vi "Voltage_laps.vi"(4 "Sweep 2":T1={"DorG_2"="", "Vvar_2_start"=0.0, "Vvar_2_step"=0.0, "Vvar_2_Stop"=0.0, "Vvar_0_stop 2"=0.0, "DrainCurComp_2 2"=1e-06, "GateCurComp_2 2"=1e-06, "Vvar_2_holdtime 2"=0.0, "Vvar_2_delaytime 2"=0.0, "IntPts_2 2"=100.0, "Set Swe_2_Mode 2"="", "Sweep Spacing_2 2"=""}, 5 "Sweep 1":T2={"DorG_1"="", "Vvar_1_start"=0.0, "Vvar_1_step"=0.0, "Vvar_1_Stop"=0.0, "Vvar_0_stop"=0.0, "DrainCurComp_1"=1e-06, "GateCurComp_1"=1e-06, "Vvar_1_holdtime"=0.0, "Vvar_1_delaytime"=0.0, "IntPts_1"=100.0, "Set Swe_1_Mode"="", "Sweep Spacing_1"=""}, 6 "error in (no error)":errorcluster, 7 "Sweep 2":bool, 8 "smu_1_port":string, 9 "VISA resource name":refnum<visa-resource-name>) -> (0 "error out":errorcluster, 1 "Recorded_data":dbl[][](array[numeric]), 3 "VISA resource name out":refnum<visa-resource-name>)   [LabVIEW 2021]
panel:
  out "V Slave":string
  out "V Lead":string
  # "Single"
  # "Double"
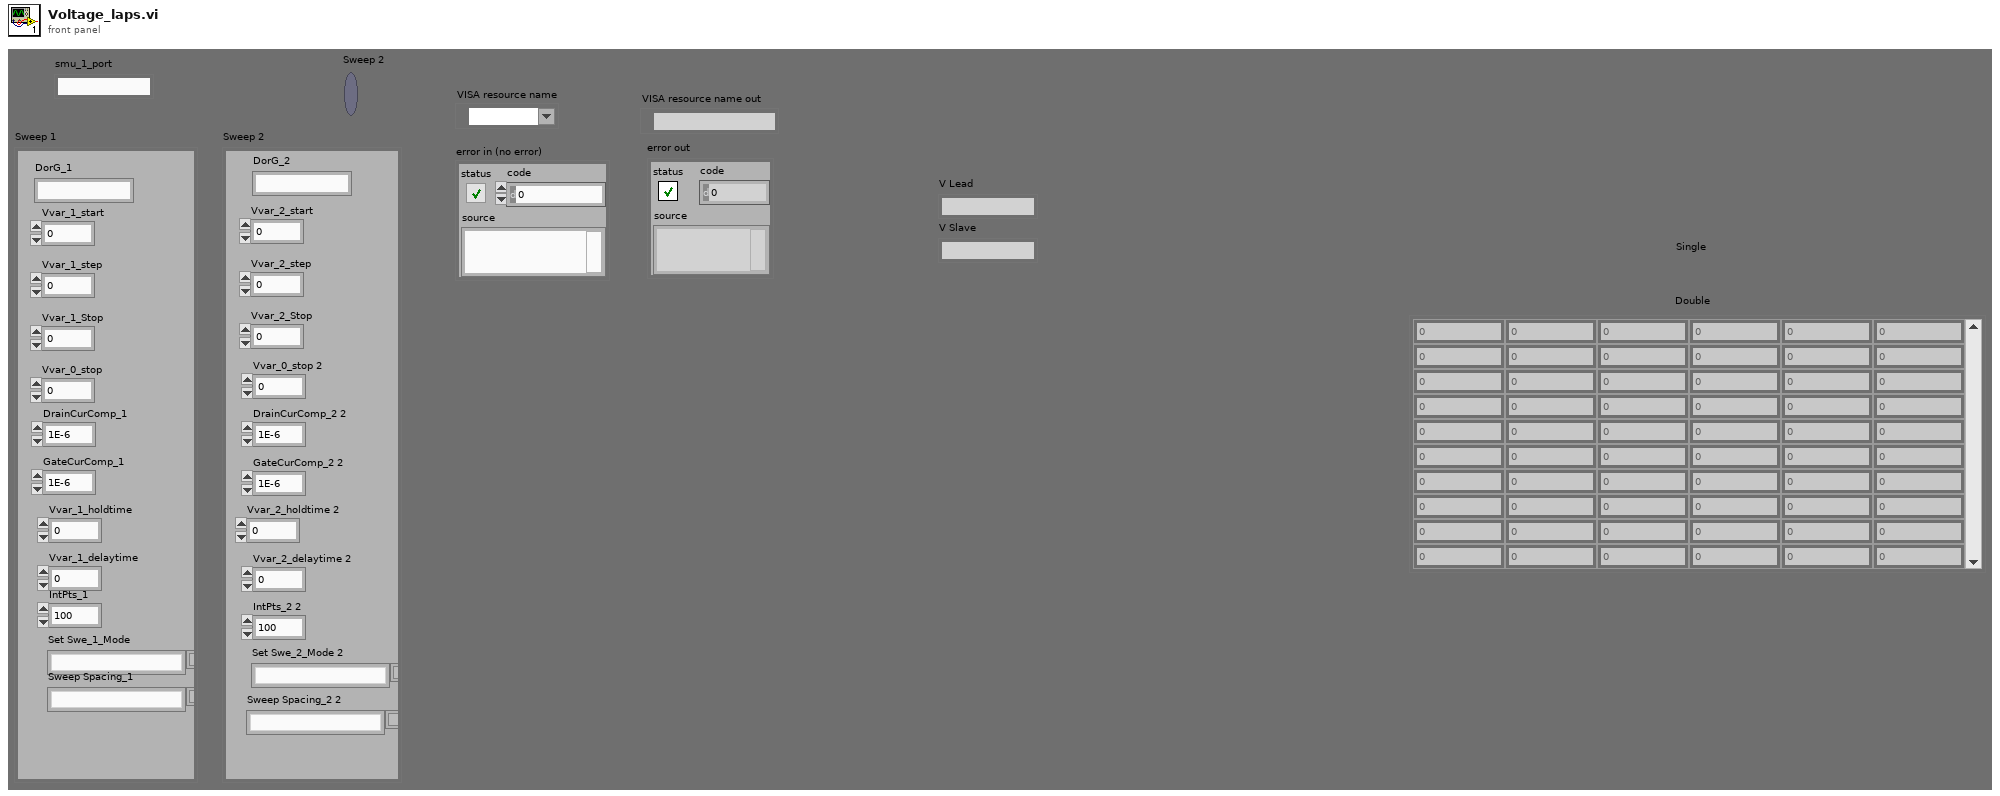
[diagram p1: front panel]
types:
  T1 = cluster{"DorG_2":string, "Vvar_2_start":dbl, "Vvar_2_step":dbl, "Vvar_2_Stop":dbl, "Vvar_0_stop 2":dbl, "DrainCurComp_2 2":dbl, "GateCurComp_2 2":dbl, "Vvar_2_holdtime 2":dbl, "Vvar_2_delaytime 2":dbl, "IntPts_2 2":dbl, "Set Swe_2_Mode 2":string, "Sweep Spacing_2 2":string}
  T2 = cluster{"DorG_1":string, "Vvar_1_start":dbl, "Vvar_1_step":dbl, "Vvar_1_Stop":dbl, "Vvar_0_stop":dbl, "DrainCurComp_1":dbl, "GateCurComp_1":dbl, "Vvar_1_holdtime":dbl, "Vvar_1_delaytime":dbl, "IntPts_1":dbl, "Set Swe_1_Mode":string, "Sweep Spacing_1":string}
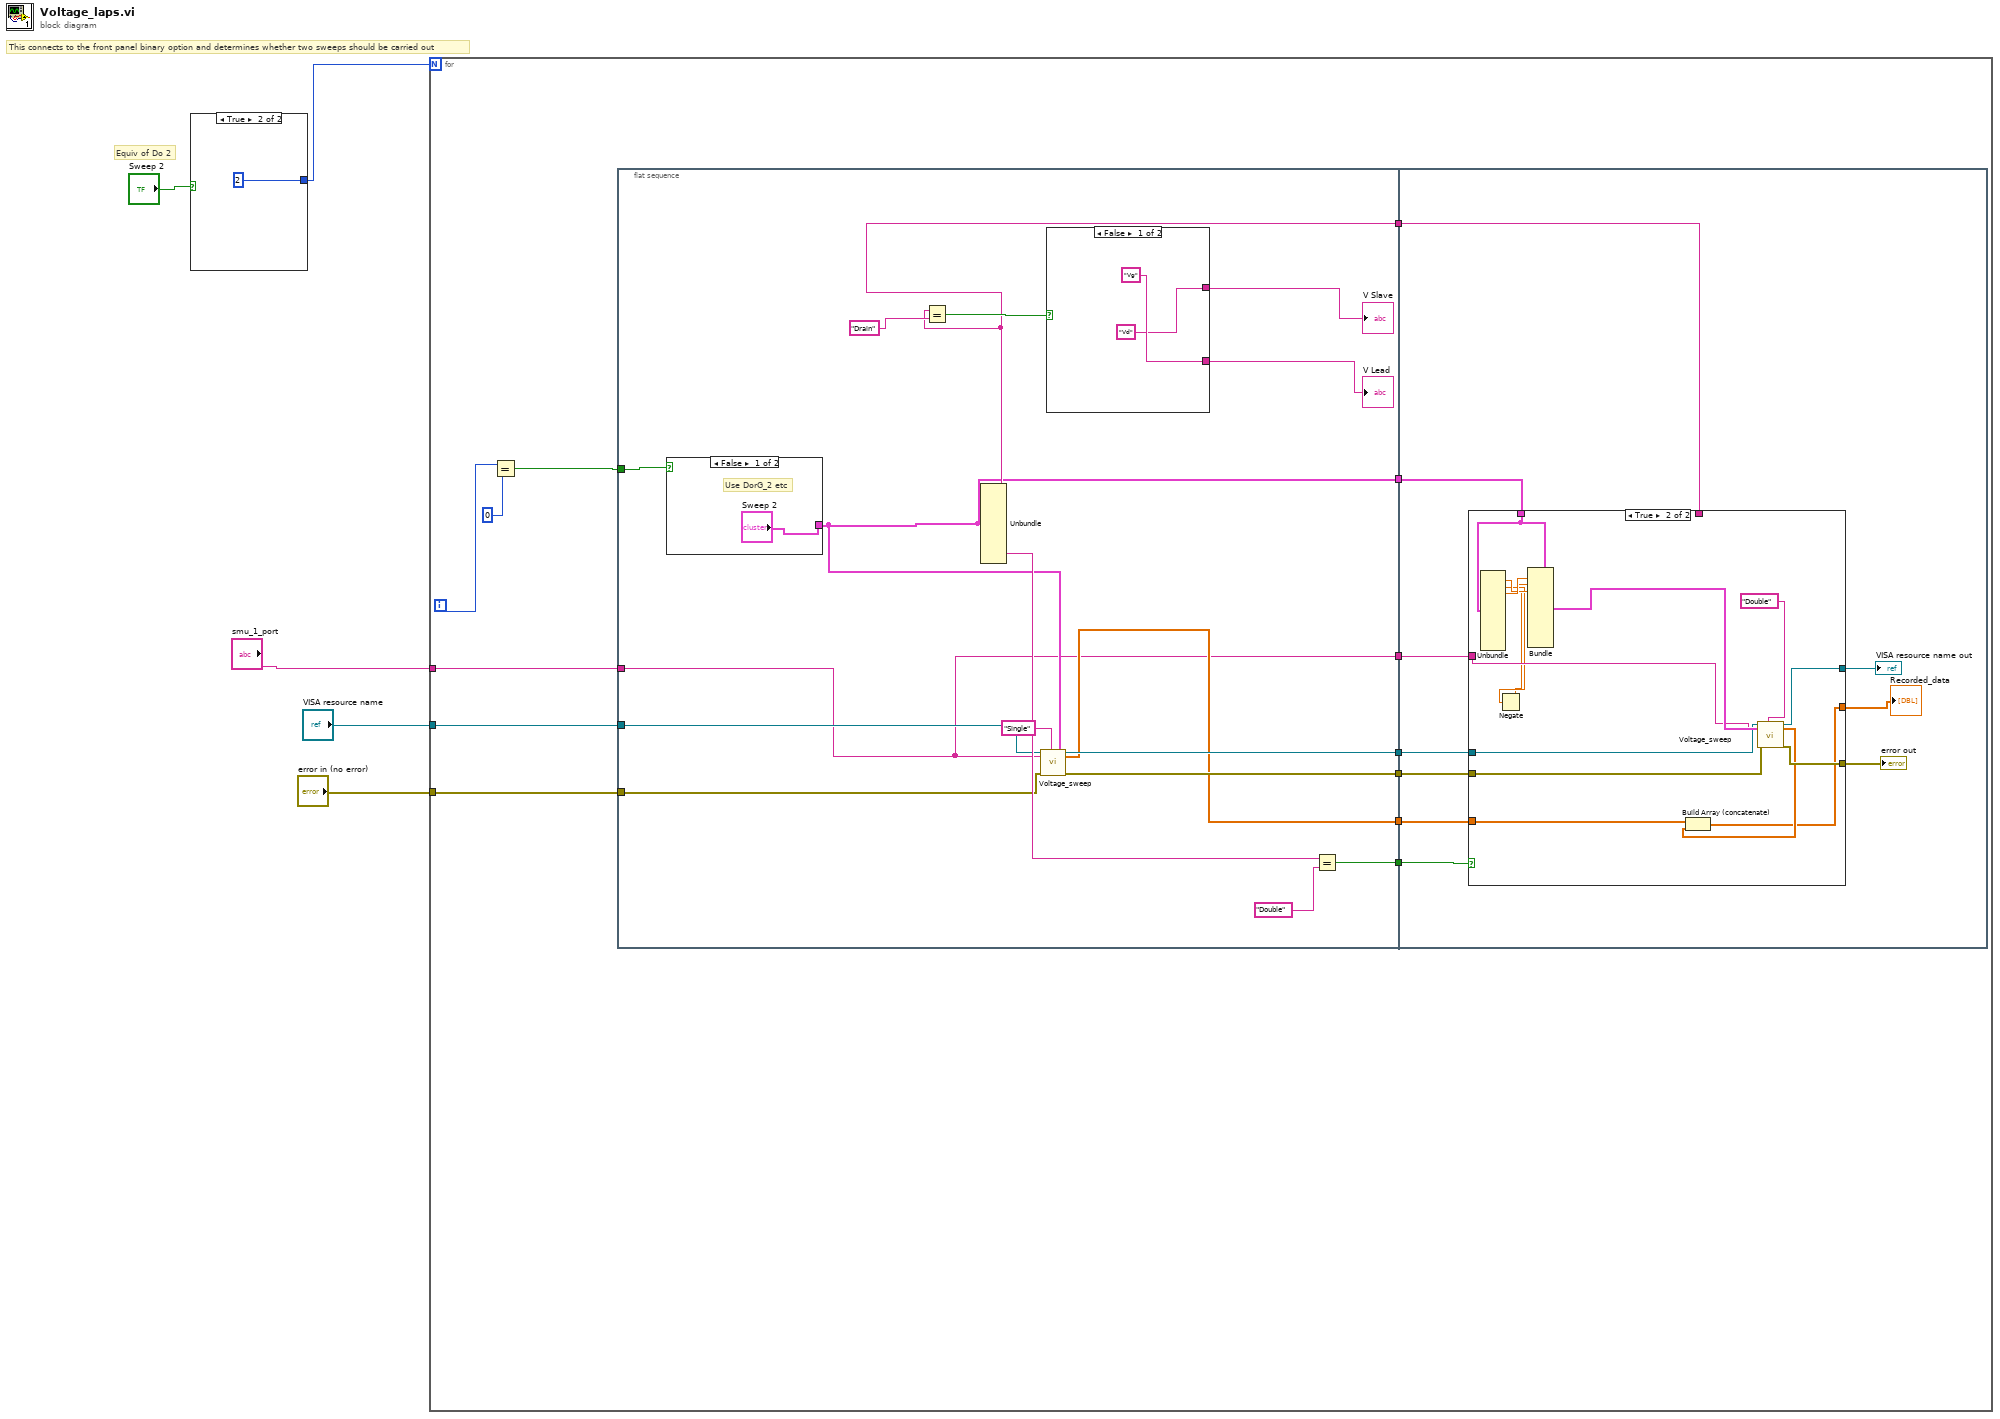
[diagram p0: block diagram]
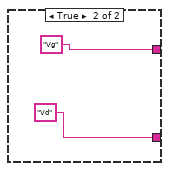
[diagram p2: hidden frame]
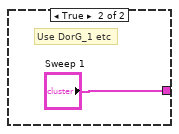
[diagram p3: hidden frame]
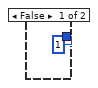
[diagram p5: hidden frame]
diagram:
  # "Equiv of Do 2"
  # "This connects to the front panel binary option and determines whether two sweeps should be carried out"
  n1 = case shown="True" "Sweep 2" {
    tunnel: [1 2] -> w4
    frame False {
    }
    frame True {
    }
  }
  n2 = for {
    N: w4 -> [_]
    tunnel: "smu_1_port" -> [w15]
    tunnel: "VISA resource name" -> [w13]
    tunnel: "error in (no error)" -> [w12]
    i -> [w20]
    n3 = Equal?(x=w20, y=0) -> (x = y?=w18:bool)
    n4 = flat-sequence {
      tunnel: w18 -> [w32]
      tunnel: [w31] -> w17
      tunnel: [w30] -> w16
      tunnel: w15 -> [w22]
      tunnel: [w28] -> w14
      tunnel: w13 -> [w27]
      tunnel: w12 -> [w26]
      tunnel: [w25] -> w11
      tunnel: [w24] -> w10
      tunnel: [w23] -> w9
      tunnel: [w22] -> w8
      tunnel: w17 -> [w53]
      tunnel: w16 -> [w52]
      tunnel: w14 -> [w50]
      tunnel: w11 -> [w49]
      tunnel: w10 -> [w48]
      tunnel: w9 -> [w45]
      tunnel: w8 -> [w44]
      frame #0 {
        n5 = case shown="False" w32 {
          tunnel: ["Sweep 2" "Sweep 1"] -> w28
          frame False {
            # "Use DorG_2 etc"
          }
          frame True {
            # "Use DorG_1 etc"
          }
        }
        n6 = Unbundle(w28) -> ("DorG_1"=w30:string, "Set Swe_1_Mode"=w29:string)  [unwired: 10 out]
        n7 = Equal?(x=w30, y="Drain") -> (x = y?=w37:bool)
        n8 = call "Voltage_sweep.vi"("VISA resource name"=w27, "smu_1_port"=w22, "error in (no error)"=w26, "Queue_name_for_multiple_streams"="Single", "Sweep 0"=w28) -> ("VISA resource name out"=w25:refnum<visa-resource-name>, "Recorded_data"=w23:dbl[][], "error out"=w24:errorcluster)  [unwired: 12 in]
        n9 = case shown="False" w37 {
          tunnel: ["Vd" "Vg"] -> w35
          tunnel: ["Vg" "Vd"] -> w36
          frame False {
          }
          frame True {
          }
        }
        "V Lead" <- w36
        "V Slave" <- w35
        n10 = Equal?(x=w29, y="Double") -> (x = y?=w31:bool)
      }
      frame #1 {
        n11 = case shown="True" w53 {
          tunnel: w52 -> [_ _]
          tunnel: w44 -> [_ w67]
          tunnel: [w54 w60] -> w51
          tunnel: w50 -> [_ w71]
          tunnel: w49 -> [w55 w66]
          tunnel: w48 -> [w56 w65]
          tunnel: [w55 w64] -> w47
          tunnel: [w56 w63] -> w46
          tunnel: w45 -> [w54 w62]
          frame False {
          }
          frame True {
            n12 = Unbundle(w71) -> ("Vvar_1_start"=w69:dbl, "Vvar_1_step"=w59:dbl, "Vvar_1_Stop"=w70:dbl)  [unwired: 9 out]
            n13 = Negate(x=w59) -> (-x=w58:dbl)
            n14 = Bundle(cluster=w71, "Vvar_1_start"=w70, "Vvar_1_step"=w58, "Vvar_1_Stop"=w69) -> (w68:T2)  [unwired: 9 in]
            n15 = call "Voltage_sweep.vi"("VISA resource name"=w66, "smu_1_port"=w67, "error in (no error)"=w65, "Queue_name_for_multiple_streams"="Double", "Sweep 0"=w68) -> ("VISA resource name out"=w64:refnum<visa-resource-name>, "Recorded_data"=w61:dbl[][], "error out"=w63:errorcluster)  [unwired: 12 in]
            n16 = Build Array (concatenate)(w62, w61) -> (w60:dbl[][])
          }
        }
        "Recorded_data" <- w51
        "error out" <- w46
        "VISA resource name out" <- w47
      }
    }
  }
